vi "Calculation State.vi"(5 "Signal Name":string, 7 "Action":T2, 8 "error in":errorcluster, 9 "Signal Values":dbl, 11 "Signal Limit Data":T1={"Nominal Value"=0.0, "Minimum"=0.0, "Maximum"=0.0, "Tolerance%"=1.0}) -> (0 "error out":errorcluster, 1 "ERROR MESSAGE":string, 2 "COMPARISON VALUE":string, 3 "In Range?":bool)   [LabVIEW 2023, in "HardwareAbstractionLayer_LVOOP.lvlib" / "Report.lvclass"]
uses:
  Report.lvclass
  Control/Calculation States.ctl
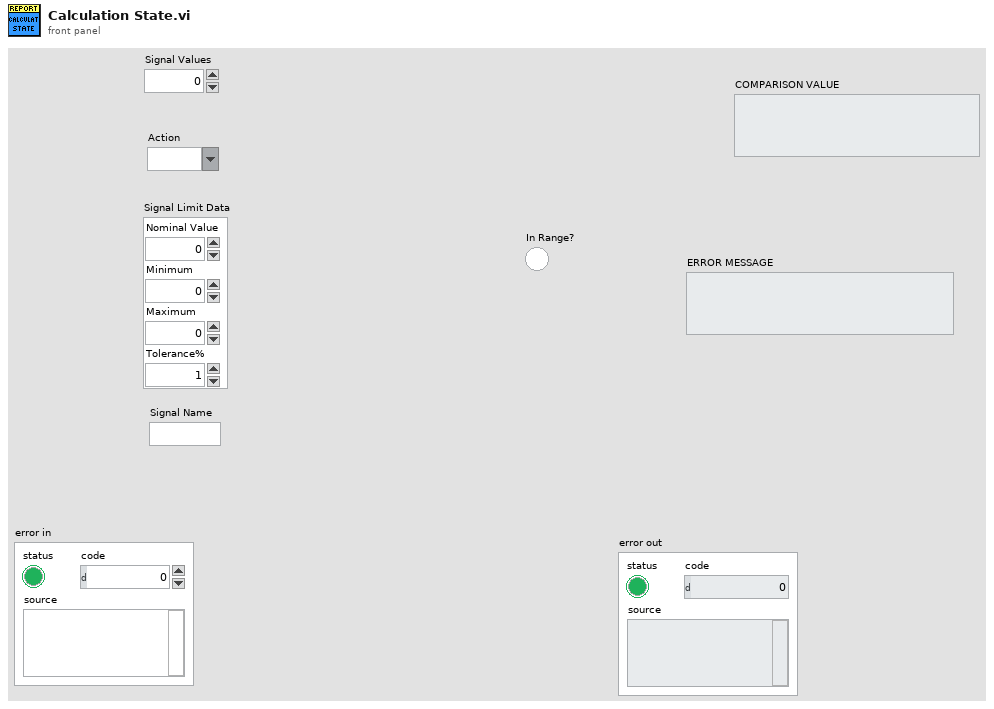
[diagram p1: front panel]
types:
  T1 = cluster{"Nominal Value":dbl, "Minimum":dbl, "Maximum":dbl, "Tolerance%":dbl}
  T2 = typedef "HardwareAbstractionLayer_LVOOP.lvlib/Report.lvclass/Calculation States.ctl" = string
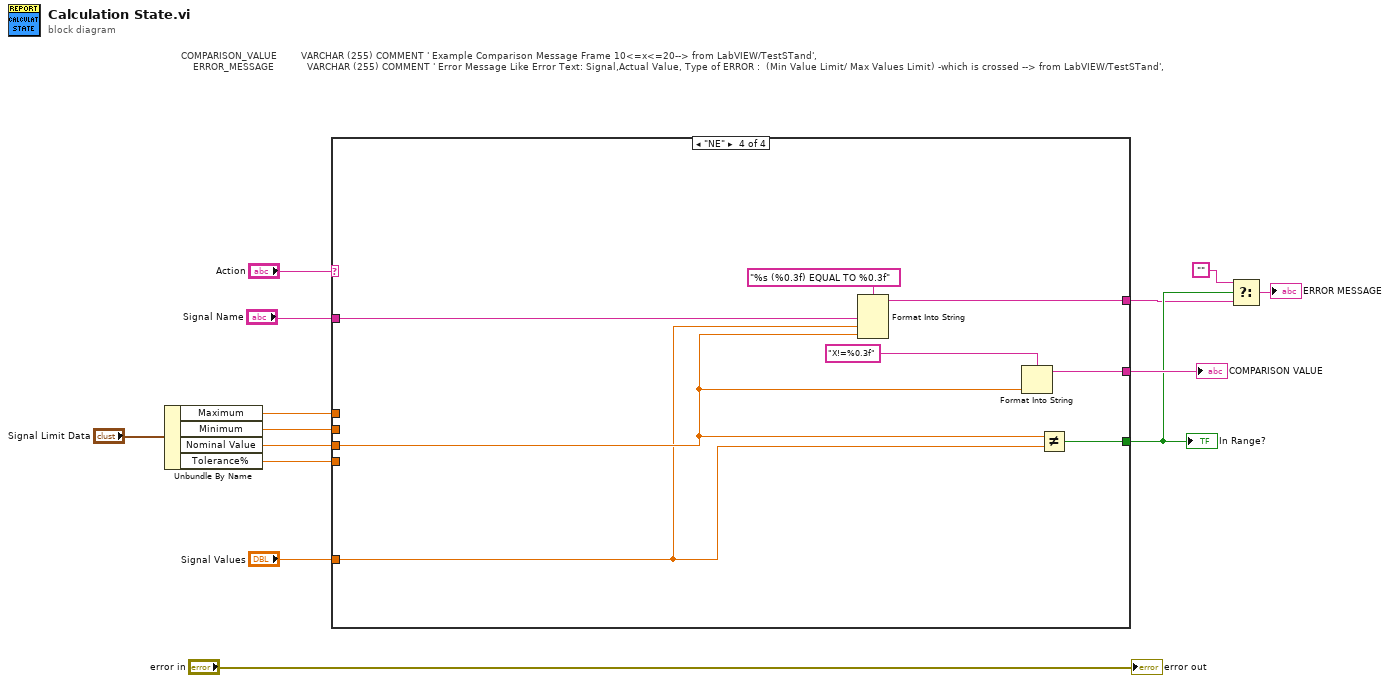
[diagram p0: block diagram]
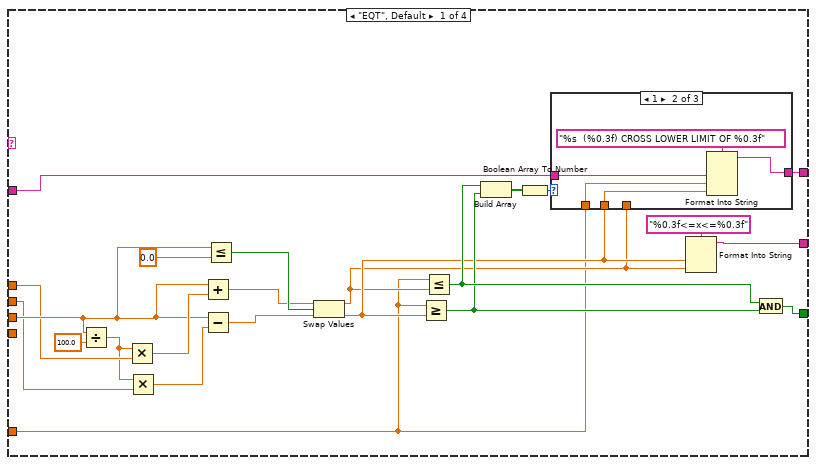
[diagram p2: hidden frame]
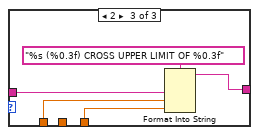
[diagram p4: hidden frame]
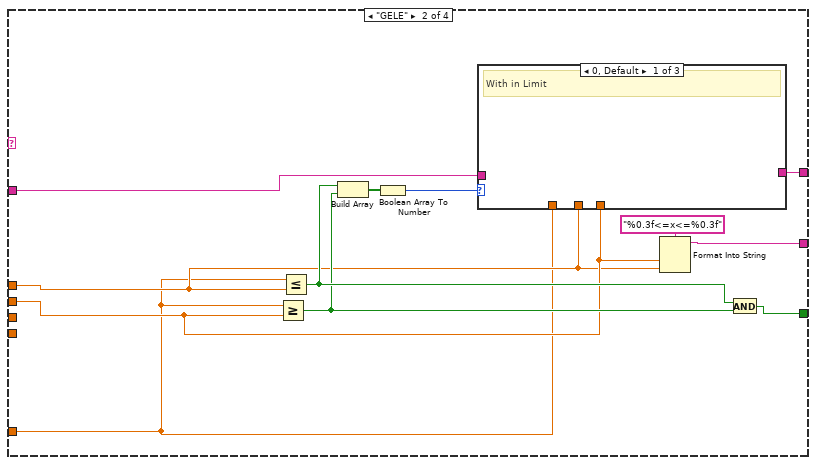
[diagram p5: hidden frame]
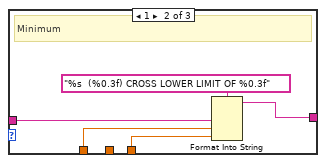
[diagram p6: hidden frame]
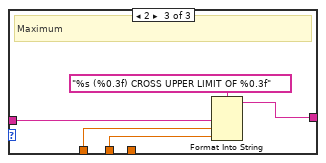
[diagram p7: hidden frame]
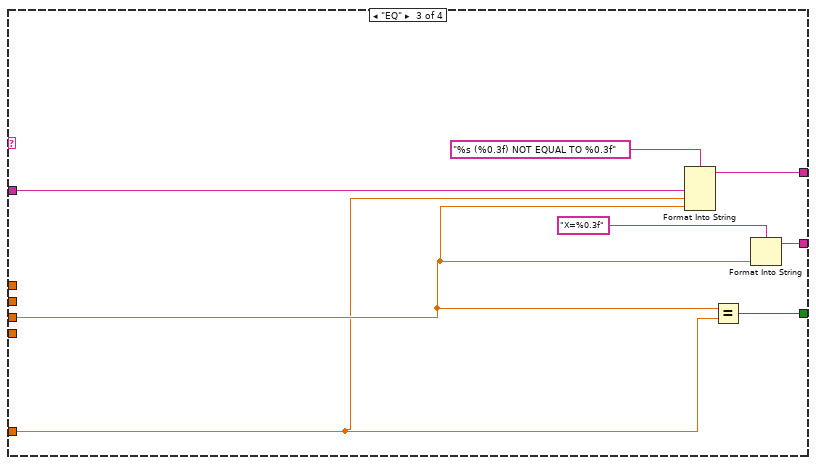
[diagram p8: hidden frame]
diagram:
  # "COMPARISON_VALUE        VARCHAR (255) COMMENT ' Example Comparison Message Frame 10<=x<=20--> from LabVIEW/TestSTand',\n    ERROR_MESSAGE           VARCHAR (255) COMMENT ' Error Message Like Error Text: Signal,Actual Value, Type of ERROR :  (Min Value Limit/ Max Values Limit) -which is crossed --> from LabVIEW/TestSTand',"
  n1 = Unbundle By Name("Signal Limit Data") -> ("Maximum"=w7:dbl, "Minimum"=w8:dbl, "Nominal Value"=w9:dbl, "Tolerance%"=w10:dbl)
  n2 = case shown="\"NE\"" "Action" {
    tunnel: w8 -> [w18 w50 _ _]
    tunnel: w7 -> [w19 w49 _ _]
    tunnel: w10 -> [_ _ _ _]
    tunnel: w9 -> [w31 _ w72 w82]
    tunnel: "Signal Values" -> [w15 w48 w70 w78]
    tunnel: [w30 w54 w77 w85] -> w4
    tunnel: [w27 w53 w75 w80] -> w6
    tunnel: "Signal Name" -> [w22 w51 w73 w79]
    tunnel: [w28 w52 w71 w81] -> w3
    frame "EQT", Default {
      n3 = Divide(x=w31, y=100.0) -> (x/y=w17:dbl)
      n4 = Multiply(x=w17, y=w19) -> (x*y=w34:dbl)
      n5 = Multiply(x=w17, y=w18) -> (x*y=w16:dbl)
      n6 = Add(x=w31, y=w34) -> (x+y=w35:dbl)
      n7 = Subtract(x=w31, y=w16) -> (x-y=w36:dbl)
      n8 = Less Or Equal?(x=w31, y=0.0) -> (x <= y?=w37:bool)
      n9 = Swap Values(12:w35, 13:w37, 14:w36) -> (1:w20:dbl, 3:w21:dbl)
      n10 = Greater Or Equal?(x=w15, y=w21) -> (x >= y?=w25:bool)
      n11 = Less Or Equal?(x=w15, y=w20) -> (x <= y?=w26:bool)
      n12 = Build Array(w26, w25) -> (w24:bool[])
      n13 = Boolean Array To Number(Boolean array=w24) -> (number=w23:u32)
      n14 = case shown="1" w23 {
        tunnel: [_ w42 w47] -> w28
        tunnel: w22 -> [_ w40 w45]
        tunnel: w21 -> [_ w39 _]
        tunnel: w20 -> [_ _ w44]
        tunnel: w15 -> [_ w38 w43]
        frame 0, Default {
          # "Withinrange"
        }
        frame 1 {
          n15 = Format Into String(format string="%s  (%0.3f) CROSS LOWER LIMIT OF %0.3f", w40, w38, w39) -> (resulting string=w42:string)  [unwired: 2 in, 1 out]
        }
        frame 2 {
          n16 = Format Into String(format string="%s (%0.3f) CROSS UPPER LIMIT OF %0.3f", w45, w43, w44) -> (resulting string=w47:string)  [unwired: 2 in, 1 out]
        }
      }
      n17 = Format Into String(format string="%0.3f<=x<=%0.3f", w21, w20) -> (resulting string=w27:string)  [unwired: 2 in, 1 out]
      n18 = And(x=w26, y=w25) -> (x .and. y?=w30:bool)
    }
    frame "GELE" {
      n19 = Greater Or Equal?(x=w48, y=w50) -> (x >= y?=w57:bool)
      n20 = Less Or Equal?(x=w48, y=w49) -> (x <= y?=w58:bool)
      n21 = Build Array(w58, w57) -> (w56:bool[])
      n22 = Boolean Array To Number(Boolean array=w56) -> (number=w55:u32)
      n23 = case shown="0, Default" w55 {
        tunnel: [_ w64 w69] -> w52
        tunnel: w51 -> [_ w62 w67]
        tunnel: w49 -> [_ _ w66]
        tunnel: w50 -> [_ w61 _]
        tunnel: w48 -> [_ w60 w65]
        frame 0, Default {
          # "With in Limit"
        }
        frame 1 {
          # "Minimum"
          n24 = Format Into String(format string="%s  (%0.3f) CROSS LOWER LIMIT OF %0.3f", w62, w60, w61) -> (resulting string=w64:string)  [unwired: 2 in, 1 out]
        }
        frame 2 {
          # "Maximum"
          n25 = Format Into String(format string="%s (%0.3f) CROSS UPPER LIMIT OF %0.3f", w67, w65, w66) -> (resulting string=w69:string)  [unwired: 2 in, 1 out]
        }
      }
      n26 = Format Into String(format string="%0.3f<=x<=%0.3f", w50, w49) -> (resulting string=w53:string)  [unwired: 2 in, 1 out]
      n27 = And(x=w58, y=w57) -> (x .and. y?=w54:bool)
    }
    frame "EQ" {
      n28 = Format Into String(format string="%s (%0.3f) NOT EQUAL TO %0.3f", w73, w70, w72) -> (resulting string=w71:string)  [unwired: 2 in, 1 out]
      n29 = Equal?(x=w72, y=w70) -> (x = y?=w77:bool)
      n30 = Format Into String(format string="X=%0.3f", w72) -> (resulting string=w75:string)  [unwired: 2 in, 1 out]
    }
    frame "NE" {
      n31 = Format Into String(format string="%s (%0.3f) EQUAL TO %0.3f", w79, w78, w82) -> (resulting string=w81:string)  [unwired: 2 in, 1 out]
      n32 = Format Into String(format string="X!=%0.3f", w82) -> (resulting string=w80:string)  [unwired: 2 in, 1 out]
      n33 = Not Equal?(x=w82, y=w78) -> (x != y?=w85:bool)
    }
  }
  "In Range?" <- w4
  "COMPARISON VALUE" <- w6
  n34 = Select(t="", s=w4, f=w3) -> (s? t:f=→"ERROR MESSAGE":string)
  "error out" <- "error in"
